vi "Get STM Reference.vi"(8 "error in (no error)":errorcluster, 9 "IP Address":u32, 10 "Port":u16=55555) -> (0 "error out":errorcluster, 4 "connection info out":T1)   [LabVIEW 2016, in "Assert API Components.lvlib" / "Log Assert Core.lvlib"]
uses:
  Log Assert Core.lvlib
  <vilib>/NI/STM/UDP/UDP Connection Info.ctl
  <vilib>/NI/STM/SubVIs/MetaDataElement.ctl
  <vilib>/NI/STM/UDP/Write Meta Data (UDP Ref).vi
  <vilib>/NI/STM/UDP/Write Meta Data (UDP Clst).vi
  <vilib>/NI/STM/NI STM.lvlib
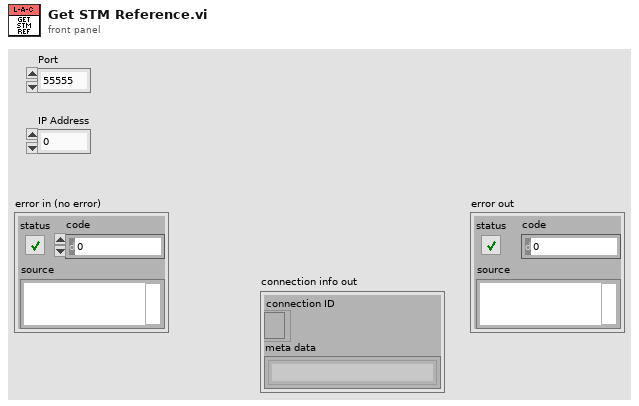
[diagram p1: front panel]
types:
  T1 = typedef "NI STM.lvlib/UDP Connection Info.ctl" = cluster{"connection ID":refnum<k16>, "meta data":T2[]}
  T2 = typedef "NI STM.lvlib/MetaDataElement.ctl" = string
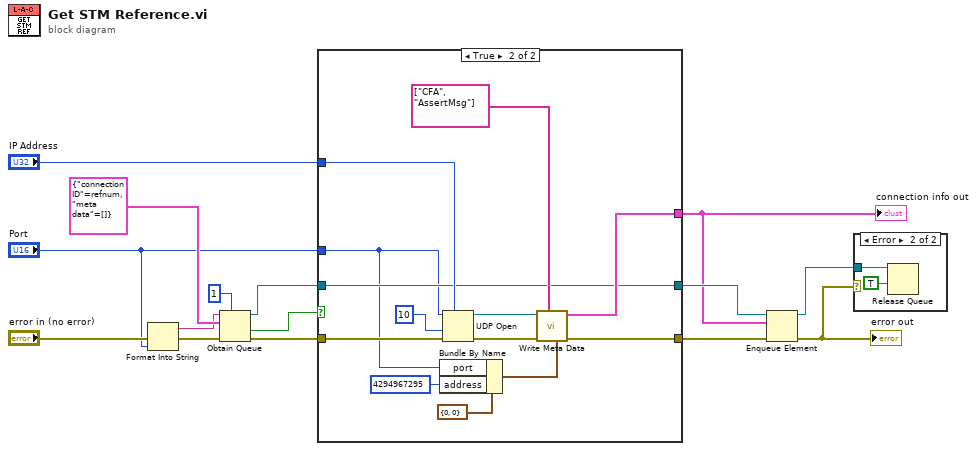
[diagram p0: block diagram]
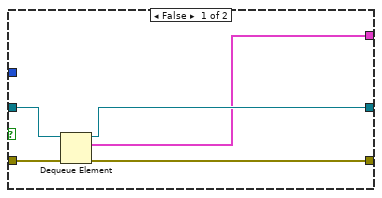
[diagram p3: hidden frame]
diagram:
  n1 = Format Into String(error in="error in (no error)", "Port") -> (resulting string=w8:string, error out=w10:errorcluster)  [unwired: 2 in]
  n2 = Obtain Queue(max queue size (-1, unlimited)=1, name (unnamed)=w8, element data type=T1 {"connection ID"=refnum, "meta data"=[]} ("connection info out"), error in (no error)=w10) -> (queue out=w5:refnum<queue>, created new?=w6:bool, error out=w12:errorcluster)  [unwired: 1 in]
  n3 = case shown="True" w6 {
    tunnel: "IP Address" -> [_ w29]
    tunnel: [w16 w28] -> w13
    tunnel: [w17 w27] -> w3
    tunnel: w12 -> [w20 w26]
    tunnel: "Port" -> [_ w22]
    tunnel: w5 -> [w19 w25]
    tunnel: [w18 w25] -> w4
    frame False {
      n4 = Dequeue Element(queue=w19, error in (no error)=w20) -> (queue out=w18:refnum<queue>, element=w17:T1, error out=w16:errorcluster)  [unwired: 1 in, 1 out]
    }
    frame True {
      n5 = Bundle By Name(cluster=cluster{"address":u32, "port":u16} {"address"=0, "port"=0} ("address"), "port"=w22, "address"=u32 4294967295) -> (w23:cluster{"address":u32, "port":u16})
      n6 = UDP Open(7:w29, 8:w26, 9:10 ("timeout ms (wait forever: -1)"), 11:w22) -> (port=w31:refnum<k16>, 0:w30:errorcluster)  [unwired: 1 in, 1 out]
      n7 = call-poly <vilib>:"Write Meta Data.vi"("address"=w23, "meta data"=T2[] ["CFA", "AssertMsg"], "error in"=w30, "connection ID"=w31) -> ("error out"=w28:errorcluster, "connection info out"=w27:T1)  [unwired: 2 in, 4 out]
    }
  }
  "connection info out" <- w3
  n8 = Enqueue Element(queue=w4, element=w3, error in (no error)=w13) -> (queue out=w2:refnum<queue>, error out=w1:errorcluster)  [unwired: 1 in, 1 out]
  "error out" <- w1
  n9 = case shown="Error" w1 {
    tunnel: w2 -> [_ w35]
    frame No Error {
    }
    frame Error {
      n10 = Release Queue(queue=w35, force destroy? (F)=TRUE) -> ()  [unwired: 1 in, 3 out]
    }
  }
